vi "test-Function-Generator-Test2.vi"(8 "error in (no error)":errorcluster) -> (0 "error out":errorcluster, 3 "All tests passed":bool)   [LabVIEW 2019]
uses:
  <vilib>/Rock Robotics/WPI/ThirdParty/JAS_Junk/TrajLib/X_Y_PAIR.ctl
  <vilib>/Rock Robotics/WPI/ThirdParty/JAS_Junk/TrajLib/FunctionGenerator_Add_Value.vi
  <vilib>/gmath/interp.llb/Search Ordered Table.vi
  <vilib>/Rock Robotics/WPI/ThirdParty/JAS_Junk/TrajLib/Trajectory_Library.lvlib
panel:
  out "Output T 7":dbl
  out "Output T 0":dbl
  out "Output T 6":dbl
  out "Output T 5":dbl
  out "Output T 4":dbl
  out "Output T 3":dbl
  out "Table Ys":dbl[](array[numeric])
  out "Table Xs":dbl[](array[numeric])
  out "Output T 2":dbl
  out "Output T 1":dbl
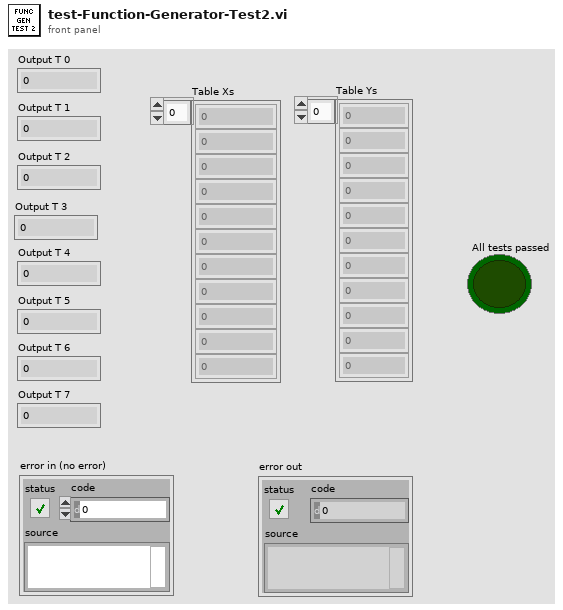
[diagram p1: front panel]
types:
  T1 = typedef "Trajectory_Library.lvlib/X_Y_PAIR.ctl" = cluster{"X":dbl, "Y":dbl}
  T2 = typedef "Trajectory_Library.lvlib/FUNCTION_GENERATOR.ctl" = cluster{"Table Xs":dbl[], "Table Ys":dbl[], "MinX":dbl, "MaxX":dbl, "ItemCount":i32}
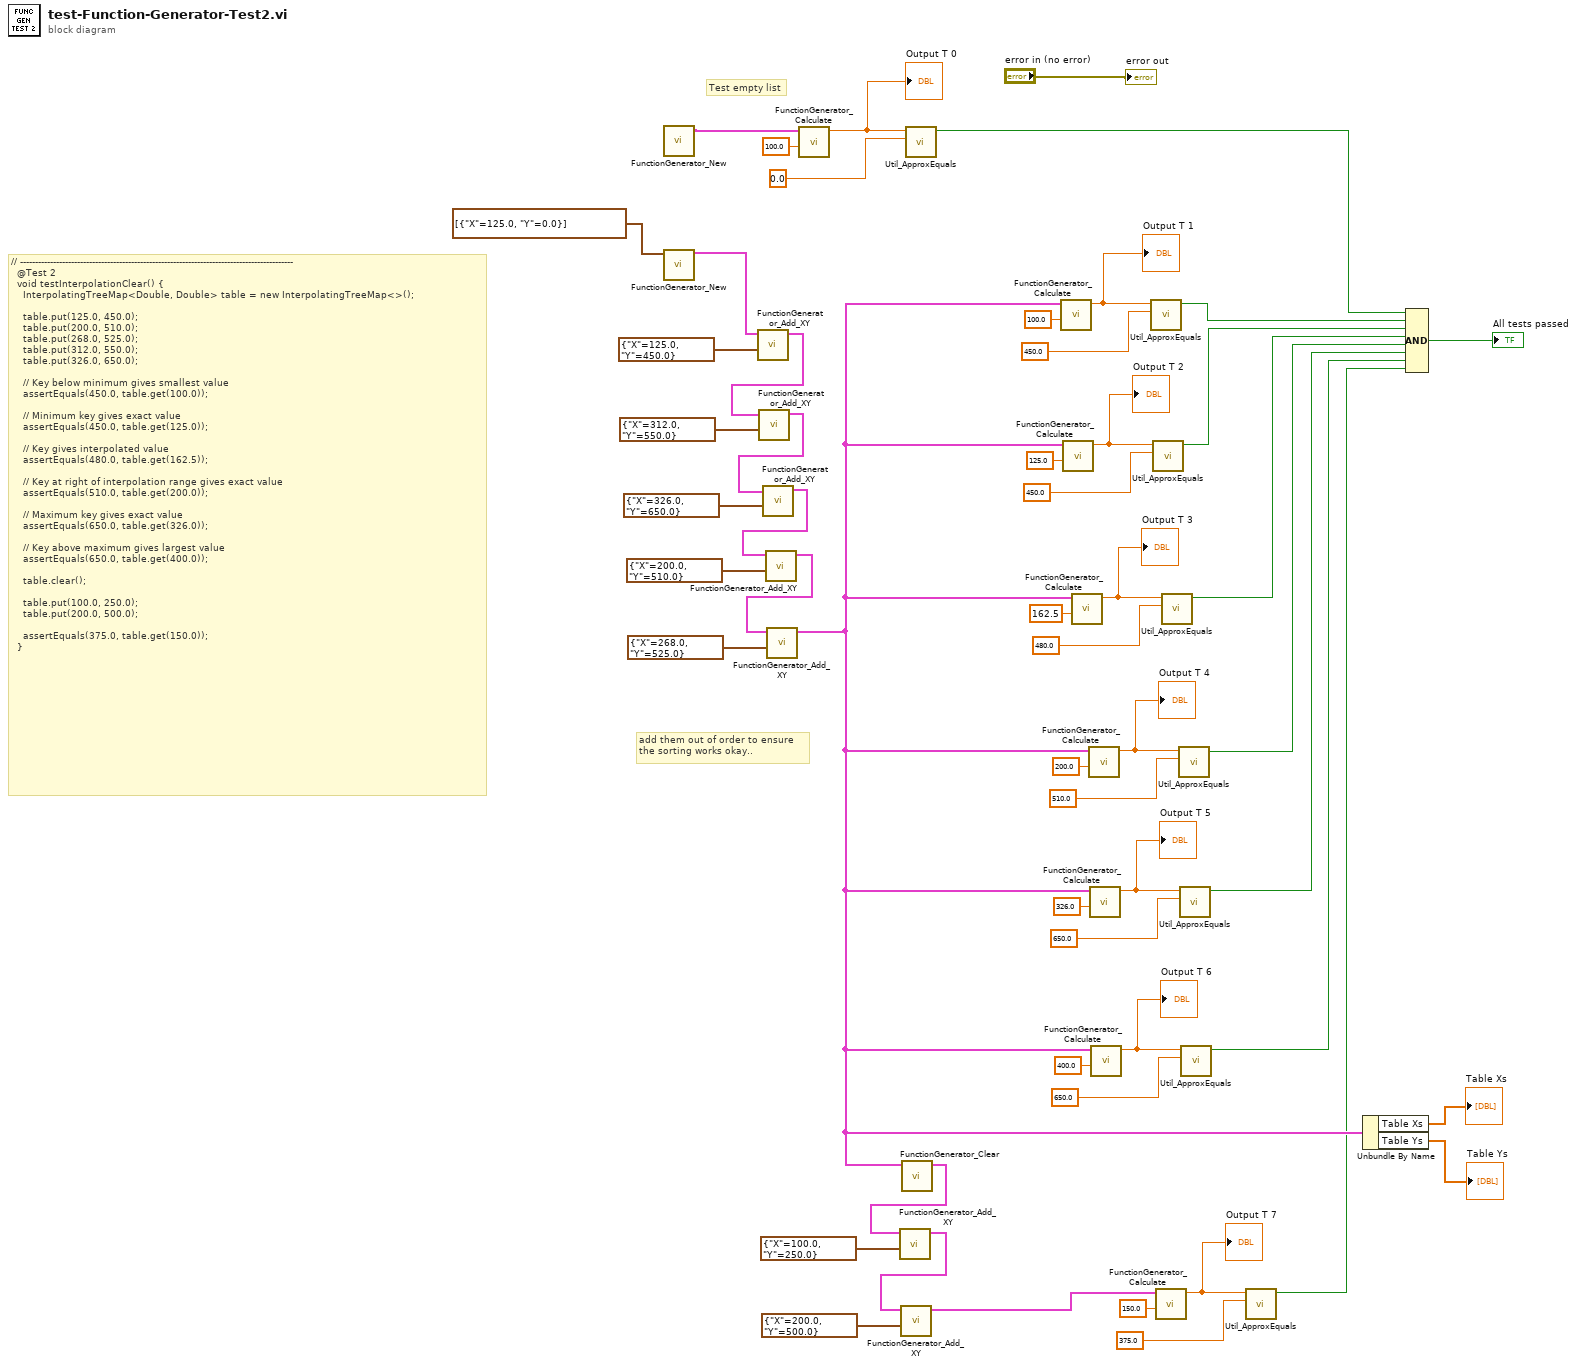
[diagram p0: block diagram]
diagram:
  # "Test empty list"
  # "add them out of order to ensure\nthe sorting works okay.."
  # "// -------------------------------------------------------------------------------------------\n  @Test 2\n  void testInterpolationClear() {\n    InterpolatingTreeMap<Double, Double> table = new InterpolatingTreeMap<>();\n\n    table.put(125.0, 450.0);\n    table.put(200.0, 510.0);\n    table.put(268.0, 525.0);\n    table.put(312.0, 550.0);\n    table.put(326.0, 650.0);\n\n    // Key below minimum gives smallest value\n    assertEquals(450.0, table.get(100.0));\n\n    // Minimum key gives exact value\n    assertEquals(450.0, table.get(125.0));\n\n    // Key gives interpolated value\n    assertEquals(480.0, table.get(162.5));\n\n    // Key at right of interpolation range gives exact value\n    assertEquals(510.0, table.get(200.0));\n\n    // Maximum key gives exact value\n    assertEquals(650.0, table.get(326.0));\n\n    // Key above maximum gives largest value\n    assertEquals(650.0, table.get(400.0));\n\n    table.clear();\n\n    table.put(100.0, 250.0);\n    table.put(200.0, 500.0);\n\n    assertEquals(375.0, table.get(150.0));\n  }"
  n1 = call <vilib>:"FunctionGenerator_New.vi"() -> ("FUNCTION_GENERATOR"=w14:T2)  [unwired: 11 in]
  n2 = call <vilib>:"FunctionGenerator_New.vi"("X Y Pairs"=T1[] [{"X"=125.0, "Y"=0.0}]) -> ("FUNCTION_GENERATOR"=w32:T2)  [unwired: 10 in]
  n3 = call <vilib>:"FunctionGenerator_Add_XY.vi"("X_Y_PAIR"=T1 {"X"=125.0, "Y"=450.0}, "in FUNCTION_GENERATOR"=w32) -> ("out FUNCTION_GENERATOR"=w47:T2)  [unwired: 9 in]
  n4 = call <vilib>:"FunctionGenerator_Add_XY.vi"("X_Y_PAIR"=T1 {"X"=312.0, "Y"=550.0}, "in FUNCTION_GENERATOR"=w47) -> ("out FUNCTION_GENERATOR"=w46:T2)  [unwired: 9 in]
  n5 = call <vilib>:"FunctionGenerator_Add_XY.vi"("X_Y_PAIR"=T1 {"X"=326.0, "Y"=650.0}, "in FUNCTION_GENERATOR"=w46) -> ("out FUNCTION_GENERATOR"=w45:T2)  [unwired: 9 in]
  n6 = call <vilib>:"FunctionGenerator_Add_XY.vi"("X_Y_PAIR"=T1 {"X"=200.0, "Y"=510.0}, "in FUNCTION_GENERATOR"=w45) -> ("out FUNCTION_GENERATOR"=w44:T2)  [unwired: 9 in]
  n7 = call <vilib>:"FunctionGenerator_Add_XY.vi"("X_Y_PAIR"=T1 {"X"=268.0, "Y"=525.0}, "in FUNCTION_GENERATOR"=w44) -> ("out FUNCTION_GENERATOR"=w10:T2)  [unwired: 9 in]
  n8 = call <vilib>:"FunctionGenerator_Calculate.vi"("Input Value"=100.0, "FUNCTION_GENERATOR"=w14) -> ("Output Value"=w13:dbl)  [unwired: 9 in]
  "Output T 0" <- w13
  n9 = call <vilib>:"FunctionGenerator_Clear.vi"("in FUNCTION_GENERATOR"=w10) -> ("out FUNCTION_GENERATOR"=w6:T2)  [unwired: 10 in]
  n10 = call <vilib>:"FunctionGenerator_Add_XY.vi"("X_Y_PAIR"=T1 {"X"=100.0, "Y"=250.0}, "in FUNCTION_GENERATOR"=w6) -> ("out FUNCTION_GENERATOR"=w7:T2)  [unwired: 9 in]
  n11 = call <vilib>:"FunctionGenerator_Add_XY.vi"("X_Y_PAIR"=T1 {"X"=200.0, "Y"=500.0}, "in FUNCTION_GENERATOR"=w7) -> ("out FUNCTION_GENERATOR"=w2:T2)  [unwired: 9 in]
  n12 = call <vilib>:"Util_ApproxEquals.vi"("Value 2"=0.0, "Value 1"=w13) -> ("ApproxEquals"=w11:bool)  [unwired: 9 in]
  n13 = call <vilib>:"FunctionGenerator_Calculate.vi"("Input Value"=100.0, "FUNCTION_GENERATOR"=w10) -> ("Output Value"=w42:dbl)  [unwired: 9 in]
  "Output T 1" <- w42
  n14 = call <vilib>:"FunctionGenerator_Calculate.vi"("Input Value"=125.0, "FUNCTION_GENERATOR"=w10) -> ("Output Value"=w35:dbl)  [unwired: 9 in]
  "Output T 2" <- w35
  n15 = call <vilib>:"FunctionGenerator_Calculate.vi"("Input Value"=162.5, "FUNCTION_GENERATOR"=w10) -> ("Output Value"=w29:dbl)  [unwired: 9 in]
  "Output T 3" <- w29
  n16 = call <vilib>:"FunctionGenerator_Calculate.vi"("Input Value"=200.0, "FUNCTION_GENERATOR"=w10) -> ("Output Value"=w26:dbl)  [unwired: 9 in]
  "Output T 4" <- w26
  n17 = call <vilib>:"FunctionGenerator_Calculate.vi"("Input Value"=326.0, "FUNCTION_GENERATOR"=w10) -> ("Output Value"=w21:dbl)  [unwired: 9 in]
  "Output T 5" <- w21
  n18 = call <vilib>:"FunctionGenerator_Calculate.vi"("Input Value"=400.0, "FUNCTION_GENERATOR"=w10) -> ("Output Value"=w18:dbl)  [unwired: 9 in]
  "Output T 6" <- w18
  n19 = call <vilib>:"Util_ApproxEquals.vi"("Value 2"=450.0, "Value 1"=w42) -> ("ApproxEquals"=w40:bool)  [unwired: 9 in]
  n20 = call <vilib>:"Util_ApproxEquals.vi"("Value 2"=450.0, "Value 1"=w35) -> ("ApproxEquals"=w36:bool)  [unwired: 9 in]
  n21 = call <vilib>:"FunctionGenerator_Calculate.vi"("Input Value"=150.0, "FUNCTION_GENERATOR"=w2) -> ("Output Value"=w3:dbl)  [unwired: 9 in]
  "Output T 7" <- w3
  n22 = call <vilib>:"Util_ApproxEquals.vi"("Value 2"=480.0, "Value 1"=w29) -> ("ApproxEquals"=w25:bool)  [unwired: 9 in]
  n23 = call <vilib>:"Util_ApproxEquals.vi"("Value 2"=510.0, "Value 1"=w26) -> ("ApproxEquals"=w24:bool)  [unwired: 9 in]
  n24 = call <vilib>:"Util_ApproxEquals.vi"("Value 2"=650.0, "Value 1"=w21) -> ("ApproxEquals"=w17:bool)  [unwired: 9 in]
  n25 = call <vilib>:"Util_ApproxEquals.vi"("Value 2"=650.0, "Value 1"=w18) -> ("ApproxEquals"=w16:bool)  [unwired: 9 in]
  n26 = call <vilib>:"Util_ApproxEquals.vi"("Value 2"=375.0, "Value 1"=w3) -> ("ApproxEquals"=w1:bool)  [unwired: 9 in]
  n27 = Unbundle By Name(w10) -> ("Table Xs"=→"Table Xs":dbl[], "Table Ys"=→"Table Ys":dbl[])
  n28 = Compound Arithmetic op=AND(w11, w40, w36, w25, w24, w17, w16, w1) -> (→"All tests passed":bool)
  "error out" <- "error in (no error)"
